vi "Write Ephemerals.vi"(8 "error in (no error)":errorcluster, 10 "Ephemerals":map{string, refnum<class "BananaPeel.lvclass">}(c390), 11 "Banana in":refnum<class "Banana.lvclass">) -> (0 "error out":errorcluster, 3 "Banana out":refnum<class "Banana.lvclass">)   [LabVIEW 2021, in "Bananas.lvlib" / "Banana.lvclass"]
uses:
  Banana.lvclass
  Banana.lvclass/Banana.ctl
  BananaPeel/BananaPeel.lvclass
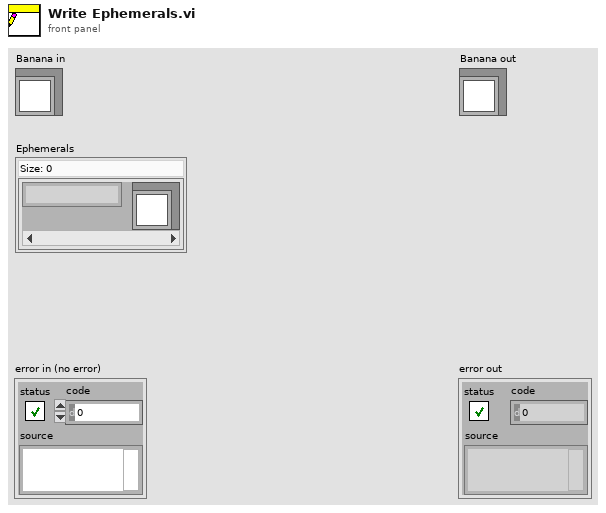
[diagram p1: front panel]
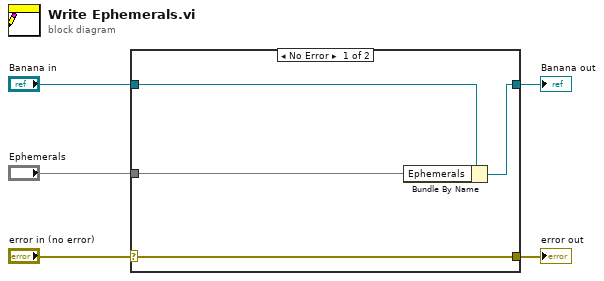
[diagram p0: block diagram]
diagram:
  n1 = case shown="No Error" "error in (no error)" {
    selector: "error in (no error)" -> [w9 w10]
    tunnel: [w9 w10] -> w4
    tunnel: [w7 w11] -> w2
    tunnel: "Banana in" -> [w8 w11]
    tunnel: "Ephemerals" -> [w6 _]
    frame No Error {
      n2 = Bundle By Name(cluster=w8, "Ephemerals"=w6) -> (w7:refnum<class "Banana.lvclass">)
    }
    frame Error {
    }
  }
  "error out" <- w4
  "Banana out" <- w2
